vi "Write.vi"(8 "error in (no error)":errorcluster, 10 "Enum Variant":variant[](array[variant]), 11 "Enum Array in":refnum<class "Enum Array.lvclass">) -> (0 "error out":errorcluster, 1 "Success?":bool, 3 "Enum Array out":refnum<class "Enum Array.lvclass">)   [LabVIEW 2020, in "Data.lvlib" / "Enum Array.lvclass"]
doc: "Write Enum Array."
uses:
  Enum Array.lvclass
  Enum Array.lvclass/Enum Array.ctl
  Enum/Enum.lvclass
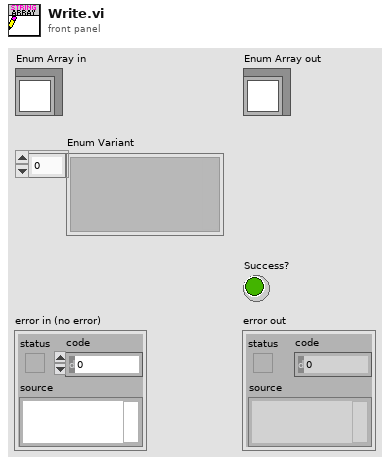
[diagram p1: front panel]
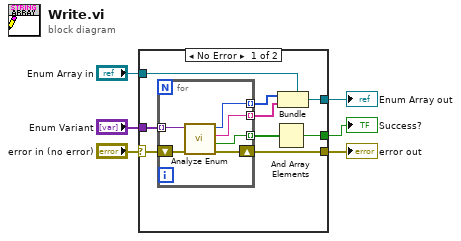
[diagram p0: block diagram]
diagram:
  n1 = case shown="No Error" "error in (no error)" {
    selector: "error in (no error)" -> [w8 w22]
    tunnel: [w7 w22] -> w5
    tunnel: [w11 w23] -> w3
    tunnel: "Enum Array in" -> [w12 w23]
    tunnel: "Enum Variant" -> [w15 _]
    tunnel: [w13 _] -> w1
    frame No Error {
      n2 = for {
        tunnel: w15 -> [w21] mode=indexing
        tunnel: [w20] -> w14 mode=indexing
        tunnel: [w19] -> w10 mode=indexing
        tunnel: [w18] -> w9 mode=indexing
        shift-right: [w16] -> w7
        shift-left: w8 -> [w17]
        n3 = call "Analyze Enum.vi"("error in (no error)"=w17, "Enum Variant"=w21) -> ("error dub"=w16:errorcluster, "Success?"=w20:bool, "Enum Alias"=w18:string, "Enum Index"=w19:u32)  [unwired: 6 in]
      }
      n4 = And Array Elements(Boolean array=w14) -> (logical AND=w13:bool)
      n5 = Bundle(cluster=w12, w10, w9) -> (w11:refnum<class "Enum Array.lvclass">)
    }
    frame Error {
    }
  }
  "error out" <- w5
  "Enum Array out" <- w3
  "Success?" <- w1
